vi "check_range.vi"(6 "Mode (Check range from Session)":T1=enum."Check range from Session", 7 "Attribute":T2={"Identifier"="", "Descriptive Name"="", "Data Type"=enum."Integer 32", "Command"="", "Access"=enum."Read/Write", "Range Table"="", "Read Callback"="", "Write Callback"="", "Supported Models"="", "Instrument Options"="", "Index"=0, "OPC Wait"=FALSE, "No Status Check"=FALSE, "Cache Only"=FALSE}, 8 "error in":errorcluster caption="error in (no error)", 10 "Value to check":dbl, 11 "VISA resource name":refnum<visa-resource-name>) -> (0 "error out":errorcluster, 3 "VISA resource name out":refnum<visa-resource-name>)   [LabVIEW 2022 SP3, in "hmp4000_rsidr_core.lvlib"]
doc: "Performs range checking if the attribute has a range table.\nRange checking mode by default is set to: based on the session settings."
uses:
  hmp4000_rsidr_core.lvlib
  type_Attribute.ctl
  type_Attribute_Data_Type.ctl
  type_ReadWriteAccess.ctl
  type_Range_CheckMode.ctl
  _type_Operation_Fgv_RangeTable.ctl
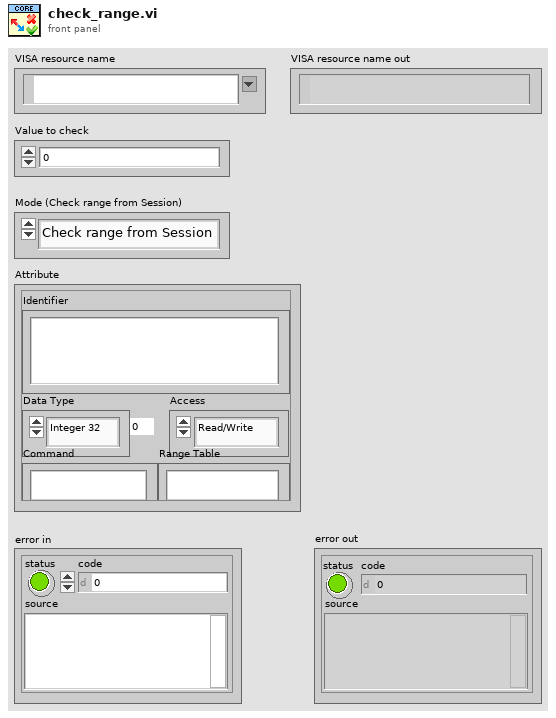
[diagram p1: front panel]
types:
  T1 = typedef "hmp4000_rsidr_core.lvlib/type_Range_CheckMode.ctl" = enum16{"Check range", "Don't check range", "Check range from Session"}
  T2 = typedef "hmp4000_rsidr_core.lvlib/type_Attribute.ctl" = cluster{"Identifier":string, "Descriptive Name":string, "Data Type":T3, "Command":string, "Access":T4, "Range Table":string, "Read Callback":string, "Write Callback":string, "Supported Models":string, "Instrument Options":string, "Index":i32, "OPC Wait":bool, "No Status Check":bool, "Cache Only":bool}
  T3 = typedef "hmp4000_rsidr_core.lvlib/type_Attribute_Data_Type.ctl" = enum16{"Integer 32", "Double", "String", "Boolean", "None", "Integer 64", "RawString"}
  T4 = typedef "hmp4000_rsidr_core.lvlib/type_ReadWriteAccess.ctl" = enum16{"Read Only", "Write Only", "Read/Write"}
  T5 = typedef "hmp4000_rsidr_core.lvlib/_type_Operation_Fgv_RangeTable.ctl" = enum16{"Initialize", "Check", "Coerce", "Get Command String", "Get Numeric Value", "Get Default Value", "Get Range Table Type"}
  T6 = typedef "hmp4000_rsidr_core.lvlib/type_Session_Data.ctl" = cluster{"IDN string":string, "Instrument FW":string, "Instr type":string, "Instr type for err. msg.":string, "Installed Options":string[], "Ignore Error Messages":string, "Logging params":variant, "OPC Timeout":i32, "VISA Timeout":i32, "STB Poll VISA Timeout":i32, "Additional Flags":i32, "Wait Before Read":i32, "Wait Before Write":i32, "Option String Flags":i32, "IO Segment Size":i64, "VISA Access Mode":T7, "Interface Type":T8, "OPC Wait Mode":T9, "Bin Float Number  Format":T10, "Bin Integer Number Format":T11, "Simulate":bool, "VXIcapable":bool, "Duplicate Session":bool, "Add LF to Write":bool, "Logging":bool, "Fast Sweep":bool, "Query Instrument Status":bool, "Check Range":bool, "Check Options":bool}
  T7 = typedef "hmp4000_rsidr_core.lvlib/type_VisaAccessMode.ctl" = u16
  T8 = typedef "hmp4000_rsidr_core.lvlib/type_InterfaceType.ctl" = enum16{"Unknown", "GPIB", "VXI", "GPIB_VXI", "ASRL", "PXI", "TCPIP", "USB", "SOCKET"}
  T9 = typedef "hmp4000_rsidr_core.lvlib/type_OPC_Wait_Mode.ctl" = enum16{"STBpolling", "STBpollingSlow", "STBpollingSuperSlow", "ServiceRequest", "OPCquery"}
  T10 = typedef "hmp4000_rsidr_core.lvlib/type_Binary_Float_Number_Format.ctl" = enum16{"Float_4_Bytes_Swapped", "Float_4_Bytes", "Double_8_Bytes_Swapped", "Double_8_Bytes"}
  T11 = typedef "hmp4000_rsidr_core.lvlib/type_Binary_Integer_Number_Format.ctl" = enum16{"Int32_4_Bytes_Swapped", "Int32_4 Bytes", "Int16_2_Bytes_Swapped", "Int16_2_Bytes"}
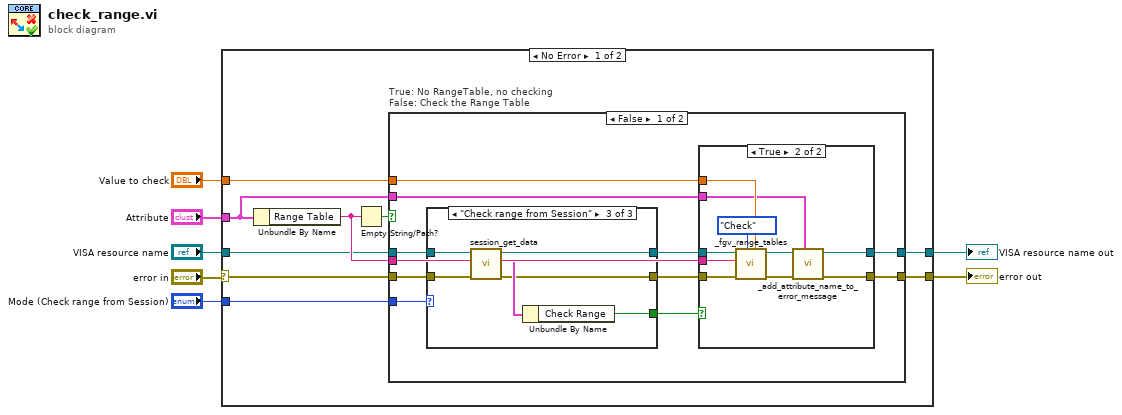
[diagram p0: block diagram]
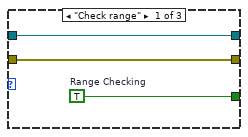
[diagram p3: hidden frame]
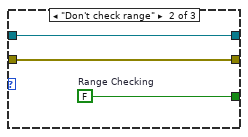
[diagram p4: hidden frame]
diagram:
  n1 = case shown="No Error" "error in" {
    selector: "error in" -> [w11 w55]
    tunnel: [w15 w55] -> w7
    tunnel: "VISA resource name" -> [w12 w54]
    tunnel: [w13 w54] -> w4
    tunnel: "Attribute" -> [w9 _]
    tunnel: "Value to check" -> [w10 _]
    tunnel: "Mode (Check range from Session)" -> [w8 _]
    frame No Error {
      n2 = Unbundle By Name(w9) -> ("Range Table"=w14:string)
      n3 = Empty String/Path?(string/path=w14) -> (empty?=w16:bool)
      n4 = case "True: No RangeTable, no checking\nFalse: Check the Range Table" shown="False" w16 {
        tunnel: w11 -> [w25 w53]
        tunnel: [w21 w53] -> w15
        tunnel: w14 -> [w26 _]
        tunnel: w12 -> [w24 w52]
        tunnel: [w18 w52] -> w13
        tunnel: w10 -> [w27 _]
        tunnel: w9 -> [w20 _]
        tunnel: w8 -> [w22 _]
        frame False {
          n5 = case shown="\"Check range from Session\"" w22 {
            tunnel: w24 -> [w42 w45 w51]
            tunnel: [w42 w45 w50] -> w19
            tunnel: [w40 w43 w46] -> w23
            tunnel: [w41 w44 w49] -> w17
            tunnel: w25 -> [w40 w43 w47]
            frame "Check range" {
              w41 = TRUE  # Range Checking
            }
            frame "Don't check range" {
              w44 = FALSE  # Range Checking
            }
            frame "Check range from Session" {
              n6 = call "session_get_data.vi"("error in"=w47, "VISA resource name"=w51) -> ("error out"=w46:errorcluster, "Session User Data out"=w48:T6, "VISA resource name out"=w50:refnum<visa-resource-name>)  [unwired: 6 in, 1 out]
              n7 = Unbundle By Name(w48) -> ("Check Range"=w49:bool)
            }
          }
          n8 = case shown="True" w17 {
            tunnel: w27 -> [_ w39]
            tunnel: w26 -> [_ w38]
            tunnel: w23 -> [w28 w37]
            tunnel: [w28 w36] -> w21
            tunnel: w20 -> [_ w35]
            tunnel: w19 -> [w29 w34]
            tunnel: [w29 w33] -> w18
            frame False {
            }
            frame True {
              n9 = call "_fgv_range_tables.vi"("Numeric Value in (0.0)"=w39, "Operation"=_type_Operation_Fgv_RangeTable."Check", "error in"=w37, "Range Table ID in"=w38, "VISA resource name"=w34) -> ("error out"=w32:errorcluster, "VISA resource name out"=w31:refnum<visa-resource-name>)  [unwired: 2 in, 3 out]
              n10 = call "_add_attribute_name_to_error_message.vi"("Attribute"=w35, "error in"=w32, "VISA resource name"=w31) -> ("error out"=w36:errorcluster, "VISA resource name out"=w33:refnum<visa-resource-name>)  [unwired: 6 in, 1 out]
            }
          }
        }
        frame True {
        }
      }
    }
    frame Error {
    }
  }
  "VISA resource name out" <- w4
  "error out" <- w7
